vi "create.vi"(5 "max (10)":dbl=10.0, 7 "min (0)":dbl, 8 "error in":errorcluster, 10 "name":string, 11 "test-channel in":refnum<class "test-channel.lvclass">) -> (0 "error out":errorcluster, 3 "test-channel out":refnum<class "test-channel.lvclass">)   [LabVIEW 2020, in "test-channel.lvclass"]
uses:
  test-channel.lvclass
  test-channel.lvclass/test-channel.ctl
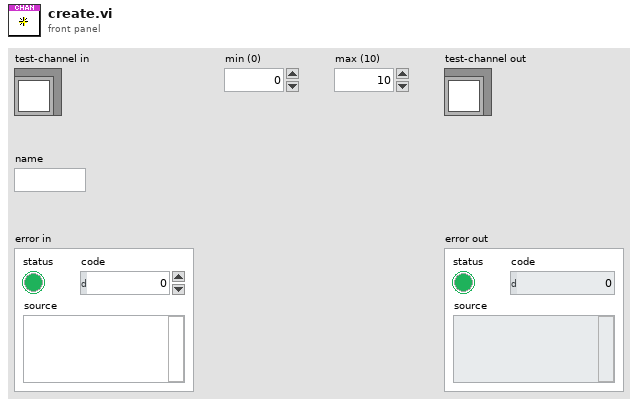
[diagram p1: front panel]
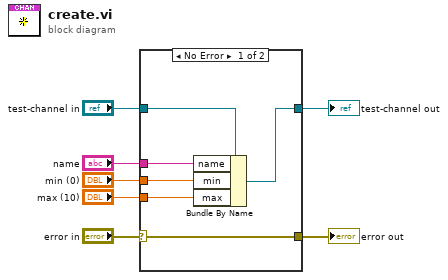
[diagram p0: block diagram]
diagram:
  n1 = case shown="No Error" "error in" {
    selector: "error in" -> [w12 w15]
    tunnel: [w12 w15] -> w6
    tunnel: [w11 w14] -> w4
    tunnel: "test-channel in" -> [w13 w14]
    tunnel: "max (10)" -> [w10 _]
    tunnel: "min (0)" -> [w9 _]
    tunnel: "name" -> [w8 _]
    frame No Error {
      n2 = Bundle By Name(cluster=w13, "name"=w8, "min"=w9, "max"=w10) -> (w11:refnum<class "test-channel.lvclass">)
    }
    frame Error {
    }
  }
  "error out" <- w6
  "test-channel out" <- w4
